vi "Add Node.vi"(8 "error in":errorcluster, 9 "Timings":T1, 10 "Node ID":u8, 11 "Node Guard in":refnum<class "Node Guard.lvclass">) -> (0 "error out":errorcluster, 3 "Node Guard out":refnum<class "Node Guard.lvclass">)   [LabVIEW 2020, in "CANopen.lvlib" / "Network Management.lvlib" / "Node Guard.lvlib" / "Node Guard.lvclass"]
uses:
  Node Guard.lvclass
  C:/Program Files/National Instruments/LabVIEW 2026/vi.lib/ActorFramework/Actor/Actor.lvclass
  Node Guard Messages/Check if Confirmed Msg/Check if Confirmed Msg.lvclass
  C:/Program Files/National Instruments/LabVIEW 2026/vi.lib/ActorFramework/Message/Message.lvclass
  <vilib>/ActorFramework/Actor/Actor.lvclass/Actor.ctl
  <vilib>/ActorFramework/Message Enqueuer/Message Enqueuer.lvclass/Message Enqueuer.ctl
  Node Guard.lvclass/Node Guard.ctl
  Node Guard Messages/Check if Confirmed Msg/Check if Confirmed Msg.lvclass/Check if Confirmed Msg.ctl
  <vilib>/ActorFramework/Message Enqueuer/Message Enqueuer.lvclass
  <vilib>/ActorFramework/Actor Framework.lvlib
  <vilib>/ActorFramework/Actor/Actor.lvclass
  <vilib>/ActorFramework/Time-Delayed Send Message/Time-Delay Override Options.ctl
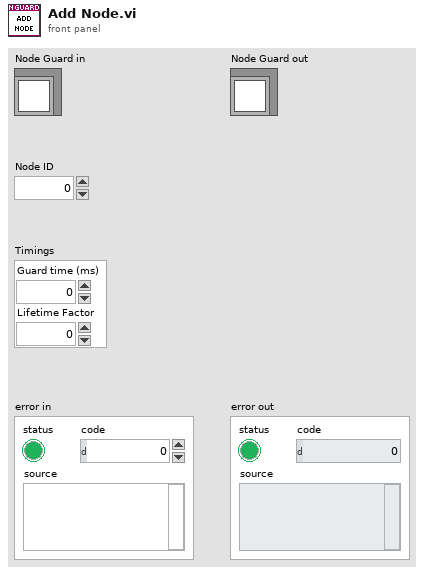
[diagram p1: front panel]
types:
  T1 = cluster{"Guard time (ms)":u16, "Lifetime Factor":u8}
  T2 = cluster{"State":u8, "Timings":cluster{"Guard time (ms)":u32, "Lifetime Factor":dbl}, "Toogle Bit":bool, "Delivery Notifier":refnum<notifier>, "Last Received Tick":u32}
  T3 = map{u8, cluster{"State":u8, "Timings":cluster{"Guard time (ms)":u16, "Lifetime Factor":u8}, "Toogle Bit":bool, "Delivery Notifier":refnum<notifier>, "Last Received Tick":u32}}
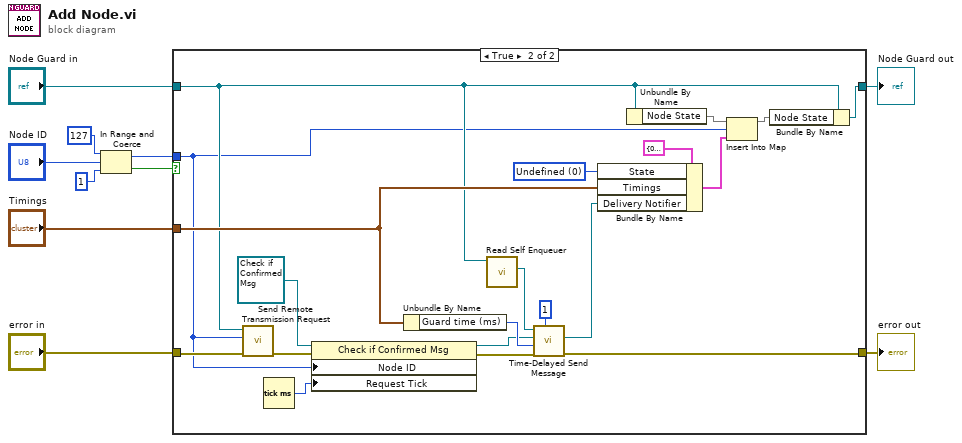
[diagram p0: block diagram]
diagram:
  n1 = In Range and Coerce(upper limit=u8 127, x="Node ID", lower limit=u8 1) -> (coerced(x)=w1:u8, In Range?=w7:bool)
  n2 = case shown="True" w7 {
    tunnel: "Node Guard in" -> [w12 w14]
    tunnel: "error in" -> [w11 w24]
    tunnel: [w11 w25] -> w4
    tunnel: [w12 w32] -> w3
    tunnel: "Timings" -> [_ w28]
    tunnel: w1 -> [_ w13]
    frame False {
    }
    frame True {
      w29 = u8 0 items=["Undefined"=0, "Stopped"=4, "Operational"=5, "Pre-operational"=127] ("State")
      n3 = call "Send Remote Transmission Request.vi"("error in"=w24, "Node ID"=w13, "Node Guard in"=w14) -> ("error out"=w21:errorcluster)  [unwired: 8 in]
      n4 = Tick Count (ms)() -> (millisecond timer value=w19:u32)
      n5 = property class="Check if Confirmed Msg"(reference=refnum<class "Check if Confirmed Msg.lvclass"> refnum ("CANopen.lvlib:Node Guard.lvlib:Check if Confirmed Msg.lvclass"), error in=w21, "Node ID"=w13, "Request Tick"=w19) -> (reference out=w22:refnum<class "Check if Confirmed Msg.lvclass">, error out=w20:errorcluster)
      n6 = Unbundle By Name(w28) -> ("Guard time (ms)"=w26:u16)
      n7 = call <vilib>:"Read Self Enqueuer.vi"("Actor"=w14) -> ("Self Enqueuer"=w17:refnum<class "Message Enqueuer.lvclass">)  [unwired: 10 in]
      n8 = call <vilib>:"Time-Delayed Send Message.vi"("# Copies (0 = infinite repeat)"=u32 1, "error in (no error)"=w20, "Milliseconds To Wait"=w26, "Message"=w22, "Message Enqueuer"=w17) -> ("error out"=w25:errorcluster, "Delivery Notifier"=w18:refnum<notifier>)  [unwired: 5 in]
      n9 = Bundle By Name(cluster=T2 {"State"=0, "Timings"={"Guard time (ms)"=0, "Lifetime Factor"=0.0}, "Toogle Bit"=FALSE, "Delivery Notifier"=refnum, "Last Received Tick"=0} ("value"), "State"=w29, "Timings"=w28, "Delivery Notifier"=w18) -> (w15:T2)
      n10 = Unbundle By Name(w14) -> ("Node State"=w30:T3)
      n11 = Insert Into Map(map in=w30, key=w13, value=w15) -> (map out=w31:T3)  [unwired: 2 out]
      n12 = Bundle By Name(cluster=w14, "Node State"=w31) -> (w32:refnum<class "Node Guard.lvclass">)
    }
  }
  "Node Guard out" <- w3
  "error out" <- w4
